vi "TestMotorsForwarda.vi"(10 "Name 2":string, 11 "Name":string) -> (3 "String":string)   [LabVIEW 2013]
uses:
  Systems/DriveMotors/DriveMotors.lvclass
  Robot Global Data.vi
panel:
  in  "MotorPower":dbl(slide) scale=-1.0..1.0
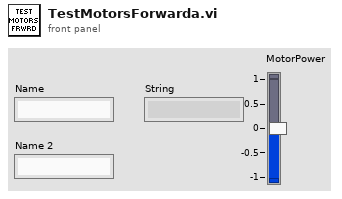
[diagram p1: front panel]
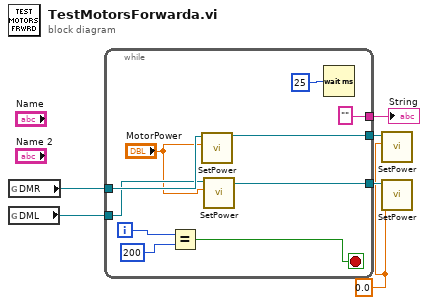
[diagram p0: block diagram]
diagram:
  w1 = 0.0 ("MotorPower")
  n1 = global read "Robot Global Data.vi" "DMR"() -> (w6:refnum<class "DriveMotors.lvclass">)
  n2 = global read "Robot Global Data.vi" "DML"() -> (w5:refnum<class "DriveMotors.lvclass">)
  n3 = while {
    tunnel: w6 -> [w12]
    tunnel: w5 -> [w11]
    tunnel: ["" ("String")] -> w4
    tunnel: [w8] -> w3
    tunnel: [w7] -> w2
    i -> [w16]
    stop <- w14 stop-if-true
    n4 = Equal?(x=w16, y=200) -> (x = y?=w14:bool)
    n5 = call-dynamic "SetPower.vi"("MotorPower"="MotorPower", "DriveMotors in"=w12) -> ("DriveMotors out"=w8:refnum<class "DriveMotors.lvclass">)  [unwired: 8 in, 1 out]
    n6 = call-dynamic "SetPower.vi"("MotorPower"="MotorPower", "DriveMotors in"=w11) -> ("DriveMotors out"=w7:refnum<class "DriveMotors.lvclass">)  [unwired: 8 in, 1 out]
    n7 = Wait (ms)(milliseconds to wait=u32 25) -> ()  [unwired: 1 out]
  }
  "String" <- w4
  n8 = call-dynamic "SetPower.vi"("MotorPower"=w1, "DriveMotors in"=w3) -> ()  [unwired: 8 in, 2 out]
  n9 = call-dynamic "SetPower.vi"("MotorPower"=w1, "DriveMotors in"=w2) -> ()  [unwired: 8 in, 2 out]
